vi "ep_Peak Search.vi"(8 "error in (no error)":errorcluster, 10 "sinc interpolation? (F)":bool, 11 "spectra points in window":T1) -> (0 "error out":errorcluster, 2 "interpolated peak frequency":dbl, 3 "interpolated peak magnitude [dB]":dbl)   [LabVIEW 2014, in "NI_EP_Motor Monitoring.lvlib"]
uses:
  <vilib>/addons/Electrical Power/Motor Monitoring/NI_EP_Motor Monitoring.lvlib
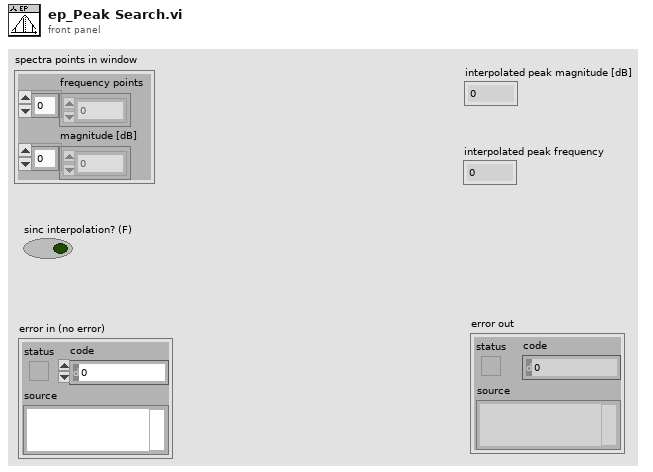
[diagram p1: front panel]
types:
  T1 = cluster{"frequency points":dbl[], "magnitude [dB]":dbl[]}
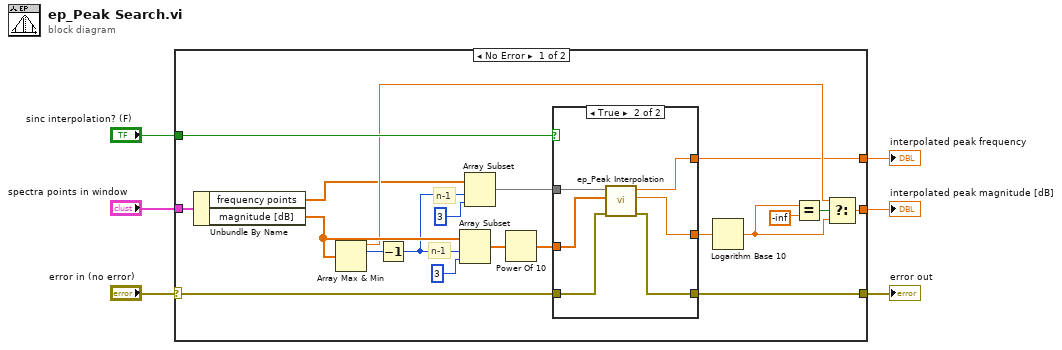
[diagram p0: block diagram]
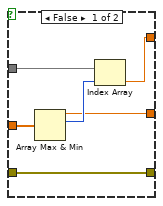
[diagram p2: hidden frame]
diagram:
  n1 = case shown="No Error" "error in (no error)" {
    selector: "error in (no error)" -> [w16 w39]
    tunnel: "spectra points in window" -> [w26 _]
    tunnel: [w15 w39] -> w4
    tunnel: [w22 _] -> w3
    tunnel: "sinc interpolation? (F)" -> [w25 _]
    tunnel: [w11 _] -> w1
    frame No Error {
      # "n-1"
      # "n-1"
      n2 = Unbundle By Name(w26) -> ("frequency points"=w13:dbl[], "magnitude [dB]"=w19:dbl[])
      n3 = Array Max & Min(array=w19) -> (max value=w14:dbl, max index (indices)=w21:i32)  [unwired: 2 out]
      n4 = Decrement(x=w21) -> (x-1=w17:i32)
      n5 = Array Subset(array=w19, index=w17, length=3) -> (w10:dbl[])
      n6 = Array Subset(array=w13, index=w17, length=3) -> (w12:dbl[])
      n7 = Power Of 10(x=w10) -> (10^x=w8:dbl[])
      n8 = case shown="True" w25 {
        tunnel: w8 -> [w31 w35]
        tunnel: w16 -> [w30 w38]
        tunnel: [w30 w37] -> w15
        tunnel: w12 -> [w29 w36]
        tunnel: [w27 w34] -> w9
        tunnel: [w28 w33] -> w11
        frame False {
          n9 = Array Max & Min(array=w31) -> (max value=w27:dbl, max index (indices)=w32:i32)  [unwired: 2 out]
          n10 = Index Array(array=w29, index=w32) -> (element=w28:dbl)
        }
        frame True {
          n11 = call <vilib>:"ep_Peak Interpolation.vi"("error in (no error)"=w38, "magnitude"=w35, "frequency [Hz]"=w36) -> ("error out"=w37:errorcluster, "fitted peak magnitude"=w34:dbl, "fitted peak frequency"=w33:dbl)  [unwired: 6 in]
        }
      }
      n12 = Logarithm Base 10(1:w9) -> (0:w7:dbl)
      n13 = Equal?(x=w7, y=-inf) -> (x = y?=w24:bool)
      n14 = Select(t=w14, s=w24, f=w7) -> (s? t:f=w22:dbl)
    }
    frame Error {
    }
  }
  "error out" <- w4
  "interpolated peak magnitude [dB]" <- w3
  "interpolated peak frequency" <- w1
